vi "Sensitivity Calculation.vi"(8 "error in (no error)":errorcluster, 11 "Tagged Sample In":dbl[](array[numeric])) -> (0 "error out":errorcluster, 3 "Tagged Sample Out":dbl[](array[numeric]))   [LabVIEW 2013]
uses:
  Data Access Objects/Metadata/Persistant DAO Actions.ctl
  Data Access Objects/Sensors/Sensor DAO Class.lvclass/Sensor DAO Class.ctl
  Data Access Objects/Sensors/Sensor List Class.lvclass
  Data Access Objects/Sensors/Sensor DAO Class.lvclass
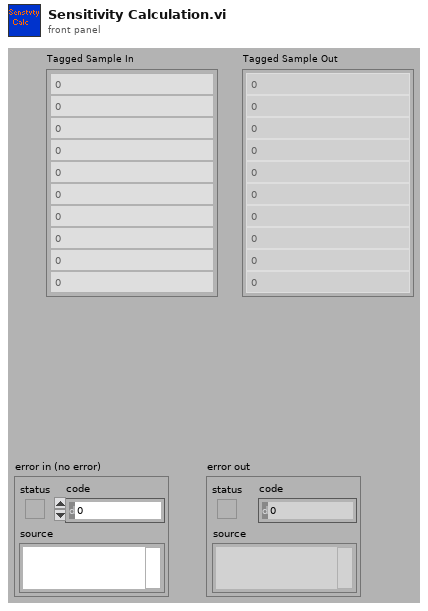
[diagram p1: front panel]
types:
  T1 = typedef "Persistant DAO Actions.ctl" = enum16{"Init", "Get", "Set", "Load", "Save"}
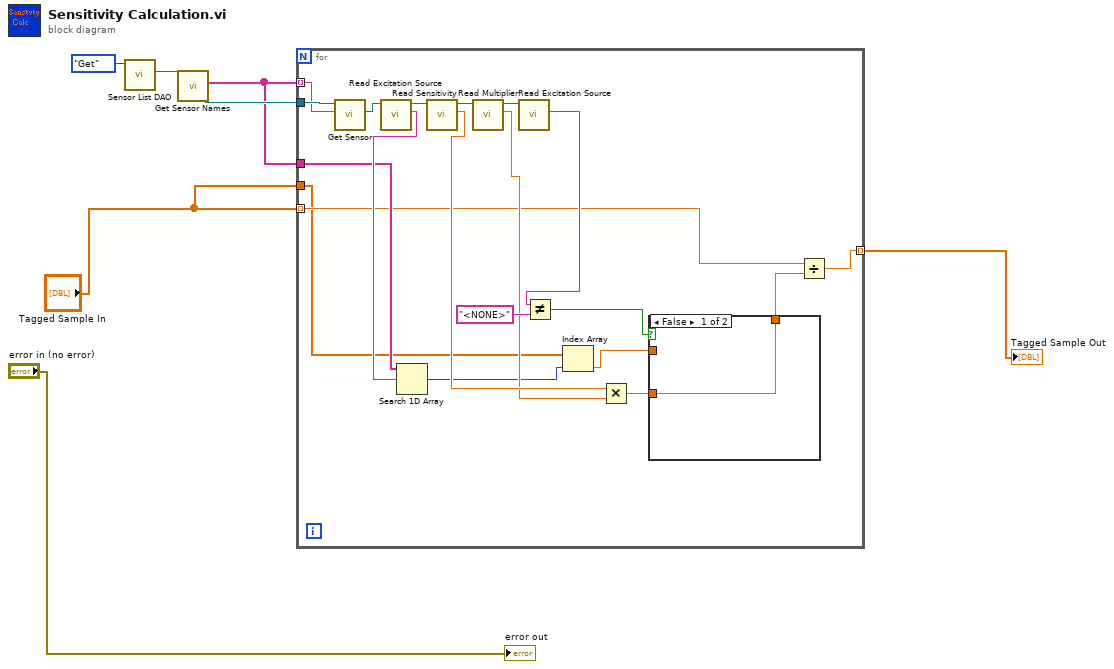
[diagram p0: block diagram]
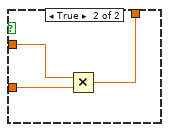
[diagram p2: hidden frame]
diagram:
  n1 = call "Sensor List DAO.vi"("Actions"=Persistant_DAO_Actions."Get") -> ("Sensor List Out"=w6:refnum<class "Sensor List Class.lvclass">)  [unwired: 8 in, 2 out]
  n2 = call "Get Sensor Names.vi"("Sensor List Class in"=w6) -> ("Names"=w4:string[], "Sensor List Class out"=w5:refnum<class "Sensor List Class.lvclass">)  [unwired: 8 in, 1 out]
  n3 = for {
    tunnel: w4 -> [w13] mode=indexing
    tunnel: w5 -> [w27]
    tunnel: w4 -> [w14]
    tunnel: "Tagged Sample In" -> [w12] mode=indexing
    tunnel: [w11] -> w3 mode=indexing
    tunnel: "Tagged Sample In" -> [w10]
    n4 = call "Get Sensor.vi"("Name"=w13, "Sensor List Class in"=w27) -> ("Sensor DAO Out"=w26:refnum<class "Sensor DAO Class.lvclass">)  [unwired: 7 in, 2 out]
    n5 = call "Read Excitation Source.vi"("Sensor DAO Class in"=w26) -> ("Excitation Source"=w25:string, "Sensor DAO Class out"=w24:refnum<class "Sensor DAO Class.lvclass">)  [unwired: 8 in, 1 out]
    n6 = Search 1D Array(1D array=w14, element=w25) -> (index of element=w9:i32)  [unwired: 1 in]
    n7 = call "Read Sensitivity.vi"("Sensor DAO Class in"=w24) -> ("Sensitivity"=w22:dbl, "Sensor DAO Class out"=w23:refnum<class "Sensor DAO Class.lvclass">)  [unwired: 8 in, 1 out]
    n8 = call "Read Multiplier.vi"("Sensor DAO Class in"=w23) -> ("Multiplier"=w17:dbl, "Sensor DAO Class out"=w21:refnum<class "Sensor DAO Class.lvclass">)  [unwired: 8 in, 1 out]
    n9 = call "Read Excitation Source.vi"("Sensor DAO Class in"=w21) -> ("Excitation Source"=w20:string)  [unwired: 8 in, 2 out]
    n10 = Not Equal?(x=w20, y="<NONE>") -> (x != y?=w18:bool)
    n11 = Index Array(array=w10, index=w9) -> (element=w8:dbl)
    n12 = Multiply(x=w22, y=w17) -> (x*y=w16:dbl)
    n13 = case shown="False" w18 {
      tunnel: [w28 w31] -> w15
      tunnel: w16 -> [w28 w30]
      tunnel: w8 -> [_ w29]
      frame False {
      }
      frame True {
        n14 = Multiply(x=w29, y=w30) -> (x*y=w31:dbl)
      }
    }
    n15 = Divide(x=w12, y=w15) -> (x/y=w11:dbl)
  }
  "Tagged Sample Out" <- w3
  "error out" <- "error in (no error)"
